vi "Write Timings Header.vi"(8 "error in (no error)":errorcluster, 11 "Save Image in":refnum<class "Save Image.lvclass">) -> (0 "error out":errorcluster, 3 "Save Image out":refnum<class "Save Image.lvclass">)   [LabVIEW 2018, in "Save Image.lvclass"]
uses:
  Save Image.lvclass
  <userlib>/gfitsio/gfitsio.lvlib
  Header/Header.lvclass
  <userlib>/gfitsio/gfitsio-write-key-string.vi
  C:/Users/observer/Desktop/SPARC4_ACS/Simulated_Header/Simulated_Header.lvclass
  Simulated_Header/Simulated_Header.lvclass
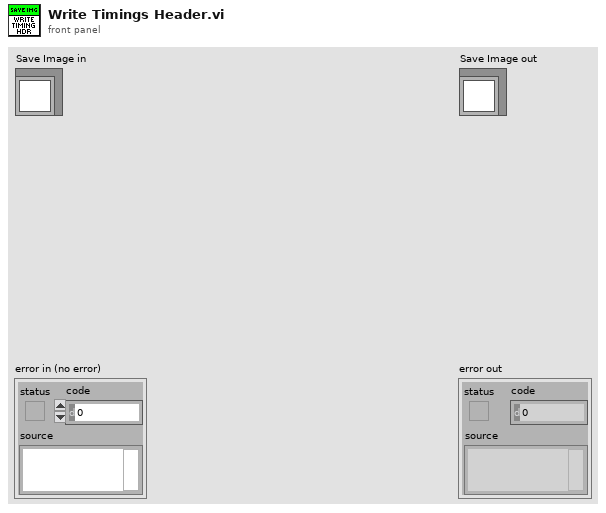
[diagram p1: front panel]
types:
  T1 = cluster{"Image Path":string, "Image Name":string, "Image Delays":string[]}
  T2 = enum16{"open", "open or create", "create or replace", "create", "open (read only)"}
  T3 = typedef "gfitsio.lvlib/gfitsio-refnum.ctl" = refnum<k1>
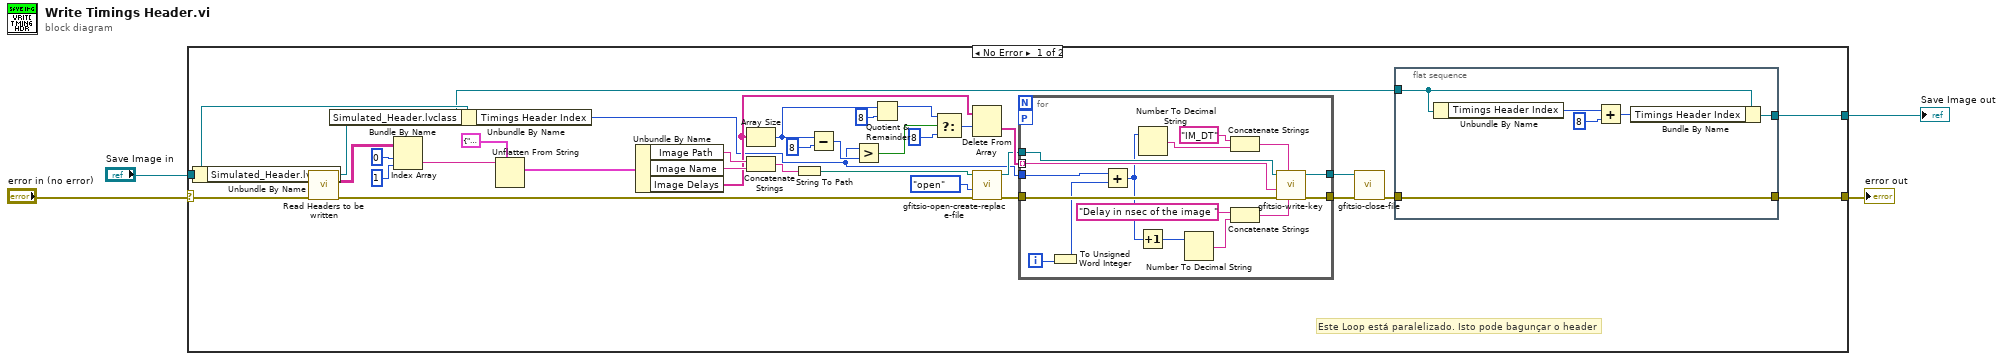
[diagram p0: block diagram]
diagram:
  n1 = case shown="No Error" "error in (no error)" {
    selector: "error in (no error)" -> [w25 w63]
    tunnel: [w17 w63] -> w3
    tunnel: [w16 w62] -> w1
    tunnel: "Save Image in" -> [w32 w62]
    frame No Error {
      # "Este Loop está paralelizado. Isto pode bagunçar o header"
      n2 = Unbundle By Name(w32) -> ("Simulated_Header.lvclass"=w26:refnum<class "Simulated_Header.lvclass">)
      n3 = call "Read Headers to be written.vi"("error in (no error)"=w25, "Header in"=w26) -> ("error out"=w20:errorcluster, "Headers to be written"=w24:string[][], "Header out"=w19:refnum<class "Header.lvclass">)  [unwired: 7 in]
      n4 = Bundle By Name(cluster=w32, "Simulated_Header.lvclass"=w19) -> (w15:refnum<class "Save Image.lvclass">)
      n5 = Index Array(array=w24, index (row)=0, index (col)=1) -> (element=w21:string)
      n6 = Unbundle By Name(w15) -> ("Timings Header Index"=w6:u16)
      n7 = Unflatten From String(type=T1 {"Image Path"="", "Image Name"="", "Image Delays"=[]} ("Image Delays Settings"), binary string=w21) -> (value=w36:T1)  [unwired: 3 in, 2 out]
      n8 = Unbundle By Name(w36) -> ("Image Path"=w30:string, "Image Name"=w29:string, "Image Delays"=w14:string[])
      n9 = Array Size(array=w14) -> (size(s)=w8:i32)
      n10 = Concatenate Strings(w30, w29) -> (w34:string)
      n11 = String To Path(string=w34) -> (path=w37:path)
      n12 = Subtract(x=w8, y=8) -> (x-y=w12:i32)
      n13 = Greater?(x=w6, y=w12) -> (0:w11:bool)
      n14 = Quotient & Remainder(x=w8, y=8) -> (x-y*floor(x/y)=w5:i32)  [unwired: 1 out]
      n15 = Select(t=w5, s=w11, f=8) -> (s? t:f=w9:i32)
      n16 = Delete From Array(array=w14, length=w9) -> (deleted portion=w31:string[])  [unwired: 1 in, 1 out]
      n17 = call <userlib>:"gfitsio-open-create-replace-file.vi"("error in (no error)"=w20, "function (open)"=T2."open", "file path (dialog if empty)"=w37) -> ("error out"=w27:errorcluster, "gfits refnum"=w28:T3)  [unwired: 6 in, 1 out]
      n18 = for {
        tunnel: w28 -> [w53]
        tunnel: [w52] -> w33
        tunnel: [w56] -> w39
        workers-P: _ -> [_]
        tunnel: w31 -> [w51] mode=indexing
        tunnel: w27 -> [w50]
        tunnel: w6 -> [w48]
        i -> [w47]
        n19 = To Unsigned Word Integer(number=w47) -> (unsigned 16bit integer=w46:u16)
        n20 = Add(x=w48, y=w46) -> (x+y=w49:u16)
        n21 = Increment(x=w49) -> (x+1=w58:u16)
        n22 = Number To Decimal String(number=w49) -> (decimal integer string=w60:string)  [unwired: 1 in]
        n23 = Number To Decimal String(number=w58) -> (decimal integer string=w54:string)  [unwired: 1 in]
        n24 = Concatenate Strings("IM_DT", w60) -> (w59:string)
        n25 = Concatenate Strings("Delay in nsec of the image " ("comment"), w54) -> (w57:string)
        n26 = call-poly <userlib>:"gfitsio-write-key.vi"("comment"=w57, "keyname"=w59, "error in (no error)"=w50, "value"=w51, "gfits refnum"=w53) -> ("error out"=w56:errorcluster, "dup gfits refnum"=w52:T3)  [unwired: 5 in]
      }
      n27 = call <userlib>:"gfitsio-close-file.vi"("error in (no error)"=w39, "gfits refnum"=w33) -> ("error out"=w18:errorcluster)  [unwired: 8 in, 1 out]
      n28 = flat-sequence {
        tunnel: w18 -> [w45]
        tunnel: [w45] -> w17
        tunnel: w15 -> [w44]
        tunnel: [w43] -> w16
        frame #0 {
          n29 = Unbundle By Name(w44) -> ("Timings Header Index"=w42:u16)
          n30 = Add(x=w42, y=8) -> (x+y=w41:i32)
          n31 = Bundle By Name(cluster=w44, "Timings Header Index"=w41) -> (w43:refnum<class "Save Image.lvclass">)
        }
      }
    }
    frame Error {
    }
  }
  "error out" <- w3
  "Save Image out" <- w1
